vi "LSMcontroller_v66_improvedwfhandling.vi"() -> ()   [LabVIEW 2015] (continued)
                                w2966 = u16 0 items=["unsigned binary", "offset binary", "2's complement"] ("data format (offset binary)")
                                n482 = Initialize Array(sgl 0.0, w2962) -> (w2969:sgl[])
                                n483 = Replace Array Subset(array=w2969, new element=sgl 1.0, index=0) -> (w2967:sgl[])
                                n484 = Reciprocal(x=w2972) -> (1/x=w2973:sgl)
                                n485 = Bundle By Name("Y"=w2967, "dt"=w2973) -> (w2964:waveform(sgl))  [unwired: 1 in]
                                n486 = call-poly <vilib>:"Analog to Digital.vi"("data format (offset binary)"=w2966, "compress digital (T)"=TRUE, "full-scale range (pk-pk)"=1.0, "resolution (16 bit)"=1, "analog waveform"=w2964) -> ("digital waveform"=w2963:digitalwaveform)  [unwired: 3 in, 3 out]
                                }
                                frame True {
                                w2979 = u16 0 items=["unsigned binary", "offset binary", "2's complement"] ("data format (offset binary)")
                                n487 = To Double Precision Float(number=w2982) -> (double precision float=w2989:dbl)
                                n488 = Initialize Array(sgl 0.0, w2982) -> (w2984:sgl[])
                                n489 = Divide(x=w2988, y=w2989) -> (x/y=w2986:dbl)
                                n490 = Round Toward +Infinity(x=w2986) -> (ceil(x): smallest int >= x=w2987:dbl)
                                n491 = Replace Array Subset(array=w2984, new element=sgl 1.0, index=0) -> (w2981:sgl[])
                                n492 = for {
                                N: w2987 -> [_]
                                tunnel: w2981 -> [w2993]
                                tunnel: [w2993] -> w2990 mode=concatenating
                                }
                                n493 = Reciprocal(x=w2991) -> (1/x=w2992:sgl)
                                n494 = Bundle By Name("Y"=w2990, "dt"=w2992) -> (w2977:waveform(sgl))  [unwired: 1 in]
                                n495 = call-poly <vilib>:"Analog to Digital.vi"("data format (offset binary)"=w2979, "compress digital (T)"=TRUE, "full-scale range (pk-pk)"=1.0, "resolution (16 bit)"=1, "analog waveform"=w2977) -> ("digital waveform"=w2976:digitalwaveform)  [unwired: 3 in, 3 out]
                                }
                                }
                                n496 = Build Array (concatenate)(w2951, w2953) -> (w2949:digitalwaveform[])
                                n497 = call "waveformsDObuffer.vi"("DO wf in"=w2949, "command"="set") -> ()  [unwired: 1 out]
                                }
                                frame 2 {
                                n498 = call "waveformsDObuffer.vi"("command"="get") -> ("DO wf out"=w2997:digitalwaveform[])  [unwired: 1 in]
                                n499 = Delete From Array(array=w2997, length=1, index=w3000) -> (deleted portion=w2995:digitalwaveform[], array with subset deleted=w2994:digitalwaveform[])
                                n500 = call "waveformsDObuffer.vi"("DO wf in"=w2994, "command"="set") -> ()  [unwired: 1 out]
                                }
                                frame 3, Default {
                                }
                                frame 0 {
                                n501 = local read "Measurement"() -> (w3003:T4)
                                n502 = To Unsigned Long Integer(number=w3003) -> (unsigned 32bit integer=w3002:u32)
                                n503 = case shown="5..7" w3002 {
                                tunnel: w3004 -> [_ w3007]
                                tunnel: [_ w3006] -> w3001
                                frame 0..4, Default {
                                }
                                frame 5..7 {
                                n504 = call "2pparameters.vi"("command"="get") -> ("params out"=w3014:T10)  [unwired: 1 in]
                                n505 = Unbundle By Name(w3014) -> ("wavdet"=w3015:bool, "sAOxy"=w3017:i32, "refwfsize"=w3018:dbl, "srate Img"=w3016:sgl)
                                n506 = call "waveformsDObuffer.vi"("command"="get") -> ("DO wf out"=w3008:digitalwaveform[])  [unwired: 1 in]
                                n507 = Index Array(array=w3008, index=w3007) -> (element=w3009:digitalwaveform)
                                n508 = case shown="True" w3015 {
                                tunnel: [w3022 w3035] -> w3012
                                tunnel: w3016 -> [w3031 w3050]
                                tunnel: w3017 -> [w3021 w3041]
                                tunnel: w3018 -> [_ w3047]
                                frame False {
                                w3025 = u16 0 items=["unsigned binary", "offset binary", "2's complement"] ("data format (offset binary)")
                                n509 = Initialize Array(sgl 0.0, w3021) -> (w3028:sgl[])
                                n510 = Replace Array Subset(array=w3028, new element=sgl 1.0, index=0) -> (w3026:sgl[])
                                n511 = Reciprocal(x=w3031) -> (1/x=w3032:sgl)
                                n512 = Bundle By Name("Y"=w3026, "dt"=w3032) -> (w3023:waveform(sgl))  [unwired: 1 in]
                                n513 = call-poly <vilib>:"Analog to Digital.vi"("data format (offset binary)"=w3025, "compress digital (T)"=TRUE, "full-scale range (pk-pk)"=1.0, "resolution (16 bit)"=1, "analog waveform"=w3023) -> ("digital waveform"=w3022:digitalwaveform)  [unwired: 3 in, 3 out]
                                }
                                frame True {
                                w3038 = u16 0 items=["unsigned binary", "offset binary", "2's complement"] ("data format (offset binary)")
                                n514 = To Double Precision Float(number=w3041) -> (double precision float=w3048:dbl)
                                n515 = Initialize Array(sgl 0.0, w3041) -> (w3043:sgl[])
                                n516 = Divide(x=w3047, y=w3048) -> (x/y=w3045:dbl)
                                n517 = Round Toward +Infinity(x=w3045) -> (ceil(x): smallest int >= x=w3046:dbl)
                                n518 = Replace Array Subset(array=w3043, new element=sgl 1.0, index=0) -> (w3040:sgl[])
                                n519 = for {
                                N: w3046 -> [_]
                                tunnel: w3040 -> [w3052]
                                tunnel: [w3052] -> w3049 mode=concatenating
                                }
                                n520 = Reciprocal(x=w3050) -> (1/x=w3051:sgl)
                                n521 = Bundle By Name("Y"=w3049, "dt"=w3051) -> (w3036:waveform(sgl))  [unwired: 1 in]
                                n522 = call-poly <vilib>:"Analog to Digital.vi"("data format (offset binary)"=w3038, "compress digital (T)"=TRUE, "full-scale range (pk-pk)"=1.0, "resolution (16 bit)"=1, "analog waveform"=w3036) -> ("digital waveform"=w3035:digitalwaveform)  [unwired: 3 in, 3 out]
                                }
                                }
                                n523 = Build Array(w3009) -> (w3006:digitalwaveform[])
                                n524 = Replace Array Subset(array=w3008, new element=w3012, index=w3007) -> (w3005:digitalwaveform[])
                                n525 = call "waveformsDObuffer.vi"("DO wf in"=w3005, "command"="set") -> ()  [unwired: 1 out]
                                }
                                }
                                }
                                }
                              }
                              frame #10 {
                                n526 = local read "Meastab"() -> (w3067:enum32{"X-Y Image", "Linescan", "Timetrace"})
                                n527 = property on="refwf" class="Ring (strict)"() -> ("RingText.Text"=w3064:string)  [unwired: 2 in, 2 out]
                                n528 = case shown="\"Timetrace\"" w3067 {
                                tunnel: [w3069 w3070] -> w3068
                                frame "X-Y Image", Default {
                                n529 = local read "Sampling rate"() -> (w3069:dbl)
                                }
                                frame "Timetrace" {
                                n530 = local read "srateAODOtt"() -> (w3070:dbl)
                                }
                                }
                                n531 = call "waveformsAObuffer.vi"("command"="get") -> ("AO wf out"=w3055:waveform(dbl)[])  [unwired: 1 in]
                                n532 = local read "wavdet"() -> (w3065:bool)
                                n533 = call "waveformsDObuffer.vi"("command"="get") -> ("DO wf out"=w3059:digitalwaveform[])  [unwired: 1 in]
                                n534 = call "correctwaveformsizetemp.vi"("new sampling frequency (Hz)"=w3068, "start"=TRUE, "reference waveforms to"=w3064, "Analog waveforms in"=w3055, "stop"=FALSE, "Digital waveforms in"=w3059) -> ("analog wf out"=w3061:waveform(dbl)[], "Digital wf out"=w3063:digitalwaveform[], "measpoints"=w3066:i32)
                                n535 = call "GetNumCamFramesv2.vi"("Digital Waveform Graph"=w3063) -> ("Numeric"=w3062:i32)  [unwired: 10 in]
                                n536 = call "waveformsDObuffer.vi"("DO wf in"=w3063, "command"="set") -> ()  [unwired: 1 out]
                                n537 = call "waveformsAObuffer.vi"("AO wf in"=w3061, "command"="set") -> ()  [unwired: 1 out]
                                n538 = local write "Total Camera Frames"(w3062) -> ()
                                n539 = case shown="True" w3065 {
                                tunnel: w3066 -> [_ w3071]
                                frame False {
                                }
                                frame True {
                                n540 = local write "# of frames"(w3071) -> ()
                                }
                                }
                              }
                            }
                          }
                          frame #6 {
                            # "Disabled for conversion to 64 bit"
                            n541 = disable-structure shown="Disabled" {
                              frame Disabled {
                                n542 = local read "Measurement"() -> (w3076:T4)
                                n543 = case shown="\"Lifetime (scan)\"" w3076 {
                                frame "X-Y-t movie", Default {
                                }
                                frame "Lifetime (scan)" {
                                # "total acquisition time"
                                n544 = call "2pparameters.vi"("command"="get") -> ("params out"=w3082:T10)  [unwired: 1 in]
                                n545 = Unbundle By Name(w3082) -> ("measpoints"=w3103:i32, "avpp"=w3104:i32, "sAOxy"=w3083:i32, "srate Img"=w3105:sgl)
                                n546 = Multiply(x=w3103, y=w3104) -> (x*y=w3101:i32)
                                n547 = To Double Precision Float(number=w3083) -> (double precision float=w3088:dbl)
                                n548 = Divide(x=w3088, y=w3105) -> (x/y=w3090:dbl)
                                n549 = To Double Precision Float(number=w3101) -> (double precision float=w3086:dbl)
                                n550 = local read "min phot"() -> (w3097:u32)
                                n551 = local read "expected c/s"() -> (w3098:dbl)
                                n552 = Multiply(x=w3086, y=w3090) -> (x*y=w3084:dbl)
                                n553 = Multiply(x=w3084, y=1000.0) -> (x*y=w3089:dbl)
                                n554 = local read "Ch1 ZeroX"() -> (w3095:i32)
                                n555 = local read "truncate"() -> (w3096:u32)
                                n556 = To Long Integer(number=w3089) -> (32bit integer=w3099:i32)
                                n557 = To Long Integer(number=w3098) -> (32bit integer=w3100:i32)
                                n558 = local read "Number of Bins"() -> (w3091:u32)
                                n559 = local read "Ch1 Level"() -> (w3093:i32)
                                n560 = local read "Ch0 ZeroX"() -> (w3094:i32)
                                n561 = local write "Acquisition time"(w3099) -> ()
                                n562 = local read "Ch0 Level"() -> (w3092:i32)
                                n563 = call "lifetimeparameters.vi"("command"="get") -> ("Params out"=w3080:T19)  [unwired: 1 in]
                                n564 = Add(x=10, y=w3099) -> (x+y=w3087:i32)
                                n565 = Bundle By Name(cluster=w3080, "acq time"=w3087, "acq rate"=w3100, "# bins"=w3091, "Ch0 Level"=w3092, "Ch1 Level"=w3093, "Ch0 ZeroX"=w3094, "Ch1 ZeroX"=w3095, "min photons"=w3097, "truncate"=w3096) -> (w3079:T19)
                                n566 = local write "Acquisition rate"(w3100) -> ()
                                n567 = call "lifetimeparameters.vi"("Params in"=w3079, "command"="set") -> ()  [unwired: 1 out]
                                }
                                }
                                n568 = local read "min phot"() -> (w3074:u32)
                                n569 = Decrement(x=w3074) -> (x-1=w3075:u32)
                                n570 = To Double Precision Float(number=w3075) -> (double precision float=w3073:dbl)
                                n571 = property on="img_CH1" class="IntGraph (strict)"("ZScale.Minimum"=w3073) -> ()  [unwired: 2 in, 2 out]
                              }
                              frame Enabled {
                              }
                            }
                            n572 = local write "64bit disabled"(TRUE ("64bit disabled")) -> ()
                          }
                          frame #7 {
                            n573 = local read "Sampling rate"() -> (w3107:dbl)
                            n574 = call "calcdaqtime.vi"("sampling rate"=w3107) -> ("Calc. time per frame (ms)"=w3106:dbl)
                            n575 = local write "Calc. time per frame (ms)"(w3106) -> ()
                          }
                          frame #8 {
                            n576 = call "2pparameters.vi"("command"="get") -> ("params out"=w3118:T10)  [unwired: 1 in]
                            n577 = local read "Measurement"() -> (w3109:T4)
                            n578 = Unbundle By Name(w3118) -> ("bufferAI"=w3116:i32, "srate"=w3117:sgl)
                            n579 = To Double Precision Float(number=w3116) -> (double precision float=w3110:dbl)
                            n580 = To Double Precision Float(number=w3117) -> (double precision float=w3120:dbl)
                            n581 = case shown="\"X-Y-t movie\", Default" w3109 {
                              tunnel: [w3125 w3129] -> w3108
                              frame "X-Y-t movie", Default {
                                n582 = local read "wavdet"() -> (w3126:bool)
                                n583 = case shown="False" w3126 {
                                tunnel: [w3127 w3128] -> w3125
                                frame False {
                                w3127 = 10123 items=["Finite Samples"=10178, "Continuous Samples"=10123, "Hardware Timed Single Point"=12522] ("sample mode")
                                }
                                frame True {
                                w3128 = 10123 items=["Finite Samples"=10178, "Continuous Samples"=10123, "Hardware Timed Single Point"=12522] ("sample mode")
                                }
                                }
                              }
                              frame "X-Y-Z stack" {
                                w3129 = 10178 items=["Finite Samples"=10178, "Continuous Samples"=10123, "Hardware Timed Single Point"=12522] ("sample mode")
                              }
                            }
                            n584 = Divide(x=w3110, y=w3120) -> (x/y=w3124:dbl)
                            n585 = Multiply(x=w3124, y=2.0) -> (x*y=w3121:dbl)
                            n586 = Max & Min(x=w3121, y=10.0) -> (max(x,y)=w3111:dbl)  [unwired: 1 out]
                            n587 = call "2pparameters.vi"("command"="get") -> ("params out"=w3115:T10)  [unwired: 1 in]
                            n588 = Bundle By Name(cluster=w3115, "timeout"=w3111, "sample mode"=w3108) -> (w3112:T10)
                            n589 = call "2pparameters.vi"("Params in"=w3112, "command"="set") -> ()  [unwired: 1 out]
                          }
                          frame #9 {
                            n590 = local read "# of frames"() -> (w3130:i32)
                            n591 = call "timestamps.vi"("# of frames"=w3130, "command"="init") -> ()  [unwired: 2 in, 1 out]
                          }
                        }
                      }
                      frame #2 {
                        # "Disabled for conversion to 64 bit"
                        n592 = call "prepAO_img.vi"() -> ("Terminal Name with Device Prefix"=w3133:tag)
                        n593 = call "prepAI_img.vi"("triggersource"=w3133) -> ()  [unwired: 2 in]
                        n594 = call "prepCI_img.vi"("ArmStart.DigEdge.Src"=w3133) -> ()  [unwired: 1 in]
                        n595 = call "prepDO_img.vi"() -> ()  [unwired: 2 in]
                        n596 = disable-structure shown="Disabled" {
                          frame Disabled {
                            n597 = local read "Measurement"() -> (w3134:T4)
                            n598 = case shown="\"Lifetime (scan)\"" w3134 {
                              frame "X-Y-t movie", Default {
                              }
                              frame "Lifetime (scan)" {
                                n599 = stacked-sequence {
                                frame #0 {
                                n600 = call "PH-temp.vi"("String"="clear" ("command")) -> ()  [unwired: 2 in, 2 out]
                                n601 = call "PH-temp-raw.vi"("command"="empty") -> ()  [unwired: 1 in, 1 out]
                                }
                                frame #1 {
                                n602 = call "calib.vi"() -> ()  [unwired: 1 in]
                                }
                                frame #2 {
                                n603 = call "setup.vi"() -> ()  [unwired: 1 in]
                                }
                                }
                              }
                            }
                          }
                          frame Enabled {
                          }
                        }
                        n604 = local write "64bit disabled"(TRUE ("64bit disabled")) -> ()
                      }
                      frame #3 {
                        n605 = local read "save\ndata"() -> (w3137:bool)
                        n606 = case shown="True" w3137 {
                          tunnel: w3138 -> [_ w3142]
                          frame False {
                          }
                          frame True {
                            n607 = local read "filename prefix"() -> (w3140:string)
                            n608 = local read "data dir"() -> (w3141:path)
                            n609 = call "preparetiffs.vi"("filename prefix"=w3140, "data dir"=w3141, "timestamp"=w3142) -> ("full-filename"=w3139:string)  [unwired: 1 in]
                            n610 = local write "full-filename"(w3139) -> ()
                          }
                        }
                        n611 = call "preptempbuffers.vi"() -> ()  [unwired: 12 in]
                      }
                      frame #4 {
                        # "Disabled Thorlabs Zstage;\nneeds to be replaced by PI code"
                        n612 = local read "Measurement"() -> (w3143:T4)
                        n613 = case shown="\"X-Y-Z stack\"" w3143 {
                          frame "X-Y-t movie", Default {
                          }
                          frame "X-Y-Z stack" {
                            # "Move Z stage"
                            n614 = stacked-sequence {
                              seq-local: [w3145 _] -> [_ w3158]
                              frame #0 {
                                n615 = local read "Z-Start (um)"() -> (w3149:dbl)
                                n616 = local read "Z-end (um)"() -> (w3148:dbl)
                                n617 = local read "# of frames"() -> (w3150:i32)
                                n618 = call "calcZslice.vi"("current slice"=0, "# of Slices"=w3150, "Z-Start (um)"=w3149, "Z-end (um)"=w3148) -> ("zpos (V)"=w3146:dbl, "zpos (um)"=w3145:dbl)
                                n619 = call "moveZ_V2.vi"("Z"=w3146) -> ()
                                n620 = local write "Cal. Z"(w3145) -> ()
                              }
                              frame #1 {
                                n621 = local read "Pstart"() -> (w3157:dbl)
                                n622 = local read "Pend"() -> (w3156:dbl)
                                n623 = local read "exp?"() -> (w3155:bool)
                                n624 = local read "Z-Start (um)"() -> (w3160:dbl)
                                n625 = local read "Z0"() -> (w3161:dbl)
                                n626 = local read "Z-end (um)"() -> (w3159:dbl)
                                n627 = local read "wavelength(nm)"() -> (w3154:dbl)
                                n628 = local read "# of frames"() -> (w3153:i32)
                                n629 = call "pockelscellzstage.vi"("current slice"=0, "# of Slices"=w3153, "wavelength (nm)"=w3154, "Z0"=w3161, "exp?"=w3155, "Zstart"=w3160, "Pend"=w3156, "Pstart"=w3157, "Z"=w3158, "Zend"=w3159) -> ("T(%)"=w3151:dbl)  [unwired: 1 in]
                                n630 = property on="Laserpower \n(%)" class="Slide (strict)"("Value"=w3151) -> ()  [unwired: 2 in, 2 out]
                                n631 = property on="lpow" class="DigNum (strict)"("Value"=w3151) -> ()  [unwired: 2 in, 2 out]
                              }
                            }
                          }
                        }
                        n632 = local write "Thorlabs Zstage disabled"(TRUE ("64bit disabled")) -> ()
                      }
                      frame #5 {
                        n633 = flat-sequence {
                          frame #0 {
                            n634 = call "2pparameters.vi"("command"="get") -> ("params out"=w3163:T10)  [unwired: 1 in]
                            n635 = Unbundle By Name(w3163) -> ("autoshutter"=w3164:bool)
                            n636 = case shown="True" w3164 {
                              frame False {
                              }
                              frame True {
                                n637 = call "shuttercontrol.vi"("command"="open") -> ()  [unwired: 1 in, 1 out]
                              }
                            }
                          }
                          frame #1 {
                            n638 = call "2pparameters.vi"("command"="get") -> ("params out"=w3168:T10)  [unwired: 1 in]
                            n639 = Tick Count (ms)() -> (millisecond timer value=w3167:u32)
                            n640 = Bundle By Name(cluster=w3168, "starttick"=w3167) -> (w3166:T10)
                            n641 = call "2pparameters.vi"("Params in"=w3166, "command"="set") -> ()  [unwired: 1 out]
                          }
                        }
                      }
                      frame #6 {
                        n642 = local read "Measurement"() -> (w3171:T4)
                        n643 = case shown="\"Lifetime (scan)\"" w3171 {
                          frame "X-Y-t movie" {
                            n644 = flat-sequence {
                              frame #0 {
                                n645 = call "runAI_img.vi"() -> ()  [unwired: 12 in]
                                n646 = call "runCI.vi"() -> ()  [unwired: 12 in]
                                n647 = call "runDO_img.vi"() -> ()  [unwired: 12 in]
                              }
                              frame #1 {
                                n648 = call "runAO_img.vi"() -> ()  [unwired: 12 in]
                              }
                            }
                          }
                          frame "Lifetime (scan)" {
                            # "Disabled for conversion to 64 bit"
                            n649 = disable-structure shown="Disabled" {
                              frame Disabled {
                                n650 = flat-sequence {
                                frame #0 {
                                n651 = call "runLT_img.vi"() -> ()  [unwired: 1 in]
                                n652 = call "runDO_img.vi"() -> ()  [unwired: 12 in]
                                }
                                frame #1 {
                                n653 = call "runAI_img.vi"() -> ()  [unwired: 12 in]
                                n654 = call "runCI.vi"() -> ()  [unwired: 12 in]
                                }
                                frame #2 {
                                n655 = call "runAO_img.vi"() -> ()  [unwired: 12 in]
                                }
                                }
                              }
                              frame Enabled {
                              }
                            }
                            n656 = local write "64bit disabled"(TRUE ("64bit disabled")) -> ()
                          }
                          frame "X-Y-Z stack", Default {
                          }
                        }
                      }
                      frame #7 {
                        # "Disabled for conversion to 64 bit"
                        n657 = while {
                          i -> [w3200]
                          stop <- w3197 stop-if-true
                          n658 = local read "Exit"() -> (w3205:bool)
                          n659 = local read "Stop"() -> (w3196:bool)
                          n660 = Or(x=w3196, y=w3205) -> (x .or. y?=w3201:bool)
                          n661 = case shown="False" w3201 {
                            tunnel: w3200 -> [w3206 _]
                            frame False {
                              n662 = stacked-sequence {
                                seq-local: [w3208 _ _ _ _ _ _] -> [_ _ _ _ _ _ w3337]
                                seq-local: [w3207 _ _ _ _ _ _] -> [_ _ _ _ _ _ w3336]
                                tunnel: w3206 -> [_ w3214 _ _ _ _ _]
                                frame #0 {
                                n663 = local read "Live"() -> (w3209:bool)
                                n664 = case shown="True" w3209 {
                                tunnel: [_ w3211] -> w3208
                                tunnel: [_ w3210] -> w3207
                                frame False {
                                }
                                frame True {
                                n665 = local read "Laserpower \n(%)"() -> (w3210:dbl)
                                n666 = local read "lpow"() -> (w3211:dbl)
                                }
                                }
                                n667 = call "preptempbuffers.vi"() -> ()  [unwired: 12 in]
                                }
                                frame #1 {
                                # "Move in Z if necessary"
                                # "Disabled Thorlabs Zstage;\nneeds to be replaced by PI code"
                                n668 = local read "Measurement"() -> (w3212:T4)
                                n669 = case shown="\"X-Y-Z stack\"" w3212 {
                                tunnel: w3214 -> [_ w3215]
                                frame "X-Y-t movie", Default {
                                }
                                frame "X-Y-Z stack" {
                                n670 = stacked-sequence {
                                seq-local: [w3216 _] -> [_ w3224]
                                tunnel: w3215 -> [w3218 w3223]
                                frame #0 {
                                n671 = local read "Z-Start (um)"() -> (w3220:dbl)
                                n672 = local read "Z-end (um)"() -> (w3219:dbl)
                                n673 = local read "# of frames"() -> (w3221:i32)
                                n674 = call "calcZslice.vi"("current slice"=w3218, "# of Slices"=w3221, "Z-Start (um)"=w3220, "Z-end (um)"=w3219) -> ("zpos (V)"=w3217:dbl, "zpos (um)"=w3216:dbl)
                                n675 = local write "Cal. Z"(w3216) -> ()
                                n676 = call "moveZ_V2.vi"("Z"=w3217) -> ()
                                }
                                frame #1 {
                                n677 = local read "Pstart"() -> (w3229:dbl)
                                n678 = local read "Pend"() -> (w3228:dbl)
                                n679 = local read "exp?"() -> (w3227:bool)
                                n680 = local read "Z-Start (um)"() -> (w3231:dbl)
                                n681 = local read "Z0"() -> (w3232:dbl)
                                n682 = local read "Z-end (um)"() -> (w3230:dbl)
                                n683 = local read "wavelength(nm)"() -> (w3226:dbl)
                                n684 = local read "# of frames"() -> (w3225:i32)
                                n685 = call "pockelscellzstage.vi"("current slice"=w3223, "# of Slices"=w3225, "wavelength (nm)"=w3226, "Z0"=w3232, "exp?"=w3227, "Zstart"=w3231, "Pend"=w3228, "Pstart"=w3229, "Z"=w3224, "Zend"=w3230) -> ("T(%)"=w3222:dbl)  [unwired: 1 in]
                                n686 = property on="Laserpower \n(%)" class="Slide (strict)"("Value"=w3222) -> ()  [unwired: 2 in, 2 out]
                                n687 = property on="lpow" class="DigNum (strict)"("Value"=w3222) -> ()  [unwired: 2 in, 2 out]
                                }
                                }
                                }
                                }
                                n688 = local write "Thorlabs Zstage disabled"(TRUE ("64bit disabled")) -> ()
                                }
                                frame #2 {
                                # "main loop"
                                n689 = for {
                                N: "avpp" -> [_]
                                i -> [w3238]
                                n690 = local read "Stop"() -> (w3236:bool)
                                n691 = local read "Exit"() -> (w3235:bool)
                                n692 = Increment(x=w3238) -> (x+1=w3237:i32)
                                n693 = Or(x=w3236, y=w3235) -> (x .or. y?=w3234:bool)
                                n694 = case shown="False" w3234 {
                                tunnel: w3237 -> [w3239 _]
                                frame False {
                                n695 = stacked-sequence {
                                seq-local: [w3240 _ _ _ _ _ _] -> [_ _ _ w3253 w3265 w3273 _]
                                tunnel: w3239 -> [w3241 _ _ _ _ _ _]
                                frame #0 {
                                n696 = local read "Live"() -> (w3240:bool)
                                n697 = case shown="True" w3240 {
                                tunnel: w3241 -> [_ w3244]
                                frame False {
                                }
                                frame True {
                                # "collect timetag for current image\nplus curent average"
                                n698 = To Single Precision Float(number=w3244) -> (single precision float=w3242:sgl)
                                n699 = Tick Count (ms)() -> (millisecond timer value=w3243:u32)
                                n700 = local write "Tick for Frame"(w3243) -> ()
                                n701 = local write "Current Average"(w3242) -> ()
                                }
                                }
                                }
                                frame #1 {
                                n702 = local read "Measurement"() -> (w3245:T4)
                                n703 = case shown="\"X-Y-Z stack\"" w3245 {
                                frame "X-Y-t movie", Default {
                                }
                                frame "X-Y-Z stack" {
                                n704 = stacked-sequence {
                                frame #0 {
                                n705 = disable-structure shown="Disabled" {
                                frame Disabled {
                                n706 = call "2pparameters.vi"("command"="get") -> ("params out"=w3247:T10)  [unwired: 1 in]
                                n707 = Unbundle By Name(w3247) -> ("autoshutter"=w3248:bool)
                                n708 = case shown="True" w3248 {
                                frame False {
                                }
                                frame True {
                                n709 = call "shuttercontrol.vi"("command"="open") -> ()  [unwired: 1 in, 1 out]
                                }
                                }
                                }
                                frame Enabled {
                                }
                                }
                                }
                                frame #1 {
                                n710 = call "runAI_img.vi"() -> ()  [unwired: 12 in]
                                n711 = call "runCI.vi"() -> ()  [unwired: 12 in]
                                n712 = call "runDO_img.vi"() -> ()  [unwired: 12 in]
                                }
                                frame #2 {
                                n713 = call "runAO_img.vi"() -> ()  [unwired: 12 in]
                                }
                                }
                                }
                                }
                                }
                                frame #2 {
                                n714 = call "collectCI_img.vi"() -> ("Avg cts/s"=w3252:dbl, "recorded samples"=w3251:i32)  [unwired: 1 out]
                                n715 = call "collectAI_img.vi"() -> ("wrap"=w3250:i32)  [unwired: 3 in]
                                n716 = local write "scol"(w3251) -> ()
                                n717 = local write "wrap"(w3250) -> ()
                                n718 = local write "Avg Counts/s"(w3252) -> ()
                                }
                                frame #3 {
                                n719 = case shown="True" w3253 {
                                frame False {
                                }
                                frame True {
                                n720 = local read "Measurement"() -> (w3254:T4)
                                n721 = case shown="\"X-Y-t movie\", Default" w3254 {
                                frame "X-Y-t movie", Default {
                                n722 = local read "ROI Type"() -> (w3255:u16)
                                n723 = case shown="0" w3255 {
                                frame 0 {
                                # "display chosen channels"
                                n724 = local read "Current Average"() -> (w3264:sgl)
                                n725 = local read "image1list"() -> (w3260:u16)
                                n726 = local read "image2list"() -> (w3263:u16)
                                n727 = To Unsigned Word Integer(number=w3263) -> (unsigned 16bit integer=w3258:u16)
                                n728 = To Unsigned Word Integer(number=w3260) -> (unsigned 16bit integer=w3259:u16)
                                n729 = call "dattoimage.vi"("image2list"=w3258, "Current Average"=w3264, "image1list"=w3259) -> ("image 2 array out"=w3262:sgl[][], "image 1 array out"=w3261:sgl[][])
                                n730 = Transpose 2D Array(2D array=w3261) -> (transposed array=w3257:sgl[][])
                                n731 = Transpose 2D Array(2D array=w3262) -> (transposed array=w3256:sgl[][])
                                n732 = local write "img_CH1"(w3257) -> ()
                                n733 = local write "img_CH2"(w3256) -> ()
                                }
                                frame 1, Default {
                                }
                                }
                                }
                                frame "Lifetime (scan)" {
                                }
                                }
                                }
                                }
                                }
                                frame #4 {
                                n734 = case shown="True" w3265 {
                                frame False {
                                }
                                frame True {
                                # "set colormaps"
                                n735 = call "misc-global.vi"("command"="get") -> ("misc out"=w3269:cluster{"Colormaps":u32[][]})  [unwired: 1 in]
                                n736 = Unbundle By Name(w3269) -> ("Colormaps"=w3268:u32[][])
                                n737 = control-ref of="img_CH1"() -> (w3272:refnum<vi>)
                                n738 = control-ref of="img_CH2"() -> (w3271:refnum<vi>)
                                n739 = Index Array(array=w3268, index (row)="Colormap") -> (element=w3267:u32[])  [unwired: 1 in]
                                n740 = property class="IntGraph (strict)"(reference=w3272, "Color Table"=w3267) -> ()  [unwired: 1 in, 2 out]
                                n741 = property class="IntGraph (strict)"(reference=w3271, "Color Table"=w3267) -> ()  [unwired: 1 in, 2 out]
                                }
                                }
                                }
                                frame #5 {
                                n742 = case shown="True" w3273 {
                                frame False {
                                }
                                frame True {
                                # "crude estimate of time per frame\n(resolution is 1 ms), not so much for\nplotting purposes, more for debugging\ncollection and processing data"
                                n743 = local read "ypixels ref"() -> (w3278:i32)
                                n744 = local read "Tick for Frame"() -> (w3279:u32)
                                n745 = Tick Count (ms)() -> (millisecond timer value=w3280:u32)
                                n746 = To Double Precision Float(number=w3278) -> (double precision float=w3277:dbl)
                                n747 = Subtract(x=w3280, y=w3279) -> (x-y=w3275:u32)
                                n748 = To Double Precision Float(number=w3275) -> (double precision float=w3276:dbl)
                                n749 = local write "Meas. time per frame (ms)"(w3275) -> ()
                                n750 = Divide(x=w3276, y=w3277) -> (x/y=w3274:dbl)
                                n751 = local write "time per line (ms)"(w3274) -> ()
                                }
                                }
                                }
                                frame #6 {
                                n752 = local read "Measurement"() -> (w3281:T4)
                                n753 = case shown="\"X-Y-Z stack\"" w3281 {
                                frame "X-Y-t movie", Default {
                                }
                                frame "X-Y-Z stack" {
                                n754 = call "2pparameters.vi"("command"="get") -> ("params out"=w3283:T10)  [unwired: 1 in]
                                n755 = Unbundle By Name(w3283) -> ("autoshutter"=w3284:bool)
                                n756 = call "stopCI_img.vi"() -> ()  [unwired: 12 in]
                                n757 = call "stopAI_img.vi"() -> ()  [unwired: 12 in]
                                n758 = case shown="True" w3284 {
                                frame False {
                                }
                                frame True {
                                n759 = call "shuttercontrol.vi"("command"="close") -> ()  [unwired: 1 in, 1 out]
                                }
                                }
                                n760 = Wait (ms)(milliseconds to wait=u32 100) -> ()  [unwired: 1 out]
                                n761 = call "stopAO_img.vi"() -> ()  [unwired: 12 in]
                                n762 = call "stopDO_img.vi"() -> ()  [unwired: 12 in]
                                }
                                }
                                }
                                }
                                }
                                frame True {
                                }
                                }
                                }
                                }
                                frame #3 {
                                n763 = local read "Measurement"() -> (w3287:T4)
                                n764 = case shown="\"Lifetime (scan)\"" w3287 {
                                frame "X-Y-t movie", Default {
                                }
                                frame "Lifetime (scan)" {
                                w3290 = u16 2 items=["Stream to disk", "Post process", "real time process"] ("Ring")
                                n765 = local read "T3R Data processing"() -> (w3291:u16)
                                n766 = Equal?(x=w3291, y=w3290) -> (x = y?=w3289:bool)
                                n767 = case shown="True" w3289 {
                                frame False {
                                }
                                frame True {
                                n768 = disable-structure shown="Disabled" {
                                frame Disabled {
                                n769 = local read "lineshift"() -> (w3294:i32)
                                n770 = call "wrapcutlifetime.vi"("lineshift"=w3294) -> ("pt3img"=w3296:u16[][], "lifetimes"=w3295:sgl[][], "okay"=w3292:bool, "# of frames"=w3293:i32)
                                n771 = case shown="True" w3292 {
                                tunnel: w3296 -> [_ w3306]
                                tunnel: w3295 -> [_ w3304]
                                tunnel: w3293 -> [_ w3300]
                                frame False {
                                }
                                frame True {
                                # "lifetime"
                                # "intensity"
                                n772 = Transpose 2D Array(2D array=w3306) -> (transposed array=w3298:u16[][])
                                n773 = Transpose 2D Array(2D array=w3304) -> (transposed array=w3305:sgl[][])
                                n774 = local write "frames recorded"(w3300) -> ()
                                n775 = local read "counts"() -> (w3299:i32)
                                n776 = Array Max & Min(array=w3298) -> (max value=w3303:u16)  [unwired: 3 out]
                                n777 = To Single Precision Float(number=w3298) -> (single precision float=w3297:sgl[][])
                                n778 = local write "img_CH2"(w3305) -> ()
                                n779 = local write "img_CH1"(w3297) -> ()
                                n780 = Quotient & Remainder(x=w3299, y=w3300) -> (floor(x/y)=→"photons/frame":i32)  [unwired: 1 out]
                                n781 = To Double Precision Float(number=w3303) -> (double precision float=w3302:dbl)
                                n782 = property on="img_CH1" class="IntGraph (strict)"("ZScale.Maximum"=w3302) -> ()  [unwired: 2 in, 2 out]
                                }
                                }
                                }
                                frame Enabled {
                                }
                                }
                                }
                                }
                                }
                                }
                                n783 = local read "save\ndata"() -> (w3288:bool)
                                n784 = case shown="True" w3288 {
                                frame False {
                                }
                                frame True {
                                n785 = local read "Current Average"() -> (w3307:sgl)
                                n786 = call "savetiffs.vi"("current average"=w3307) -> ()
                                }
                                }
                                }
                                frame #4 {
                                n787 = local read "save\ndata"() -> (w3308:bool)
                                n788 = case shown="True" w3308 {
                                frame False {
                                }
                                frame True {
                                n789 = local read "points recorded"() -> (w3310:i32)
                                n790 = call "timestamps.vi"("points recorded"=w3310, "command"="add") -> ()  [unwired: 2 in, 1 out]
                                }
                                }
                                }
                                frame #5 {
                                n791 = local read "Live"() -> (w3311:bool)
                                n792 = case shown="True" w3311 {
                                frame False {
                                }
                                frame True {
                                n793 = local read "downright"() -> (w3316:bool)
                                n794 = local read "downleft"() -> (w3318:bool)
                                n795 = local read "upright"() -> (w3314:bool)
                                n796 = local read "upleft"() -> (w3312:bool)
                                n797 = local read "down"() -> (w3317:bool)
                                n798 = local read "right"() -> (w3315:bool)
                                n799 = local read "left"() -> (w3319:bool)
                                n800 = local read "up"() -> (w3313:bool)
                                n801 = Compound Arithmetic op=OR(w3312, w3313, w3314, w3315, w3316, w3317, w3318, w3319) -> (w3320:bool)
                                n802 = case shown="True" w3320 {
                                frame False {
                                }
                                frame True {
                                n803 = stacked-sequence {
                                frame #0 {
                                n804 = local read "downright"() -> (w3322:bool)
                                n805 = local read "downleft"() -> (w3324:bool)
                                n806 = local read "BigSmall"() -> (w3321:bool)
                                n807 = local read "upright"() -> (w3326:bool)
                                n808 = local read "upleft"() -> (w3329:bool)
                                n809 = local read "down"() -> (w3325:bool)
                                n810 = local read "right"() -> (w3327:bool)
                                n811 = local read "left"() -> (w3323:bool)
                                n812 = local read "up"() -> (w3328:bool)
                                n813 = call "movestageparams.vi"("command"="get") -> ("Params out"=w3332:T20)  [unwired: 1 in]
                                n814 = Bundle By Name(cluster=w3332, "upleft"=w3329, "up"=w3328, "upright"=w3326, "right"=w3327, "downright"=w3322, "down"=w3325, "downleft"=w3324, "left"=w3323, "Bigsmall"=w3321) -> (w3333:T20)
                                n815 = call "movestageparams.vi"("Params in"=w3333, "command"="set") -> ()  [unwired: 1 out]
                                }
                                frame #1 {
                                n816 = call "movestage.vi"() -> ()  [unwired: 12 in]
                                }
                                frame #2 {
                                w3334 = FALSE ("OK Button")
                                w3335 = FALSE ("OK Button")
                                n817 = property on="down" class="Bool (strict)"("Value"=w3335) -> ()  [unwired: 2 in, 2 out]
                                n818 = property on="up" class="Bool (strict)"("Value"=w3335) -> ()  [unwired: 2 in, 2 out]
                                n819 = property on="right" class="Bool (strict)"("Value"=w3335) -> ()  [unwired: 2 in, 2 out]
                                n820 = property on="left" class="Bool (strict)"("Value"=w3335) -> ()  [unwired: 2 in, 2 out]
                                n821 = property on="upright" class="Bool (strict)"("Value"=w3334) -> ()  [unwired: 2 in, 2 out]
                                n822 = property on="downleft" class="Bool (strict)"("Value"=w3334) -> ()  [unwired: 2 in, 2 out]
                                n823 = property on="downright" class="Bool (strict)"("Value"=w3334) -> ()  [unwired: 2 in, 2 out]
                                n824 = property on="upleft" class="Bool (strict)"("Value"=w3334) -> ()  [unwired: 2 in, 2 out]
                                }
                                }
                                }
                                }
                                }
                                }
                                }
                                frame #6 {
                                n825 = local read "Live"() -> (w3338:bool)
                                n826 = case shown="True" w3338 {
                                tunnel: w3337 -> [_ w3345]
                                tunnel: w3336 -> [_ w3344]
                                frame False {
                                }
                                frame True {
                                n827 = local read "Laserpower \n(%)"() -> (w3340:dbl)
                                n828 = local read "lpow"() -> (w3339:dbl)
                                n829 = Not Equal?(x=w3339, y=w3345) -> (x != y?=w3341:bool)
                                n830 = Not Equal?(x=w3340, y=w3344) -> (x != y?=w3342:bool)
                                n831 = Or(x=w3342, y=w3341) -> (x .or. y?=w3343:bool)
                                n832 = case shown="True" w3343 {
                                tunnel: w3342 -> [_ w3349]
                                tunnel: w3341 -> [_ w3348]
                                tunnel: w3340 -> [_ w3347]
                                tunnel: w3339 -> [_ w3346]
                                frame False {
                                }
                                frame True {
                                n833 = case shown="True" w3349 {
                                tunnel: w3347 -> [_ w3352]
                                frame False {
                                }
                                frame True {
                                n834 = local read "wavelength(nm)"() -> (w3353:dbl)
                                n835 = call "setpockelscellT.vi"("wavelength(nm)"=w3353, "transmission"=w3352) -> ()  [unwired: 1 in]
                                n836 = property on="lpow" class="DigNum (strict)"("Value"=w3352) -> ()  [unwired: 2 in, 2 out]
                                }
                                }
                                n837 = case shown="True" w3348 {
                                tunnel: w3346 -> [_ w3350]
                                frame False {
                                }
                                frame True {
                                n838 = local read "wavelength(nm)"() -> (w3351:dbl)
                                n839 = call "setpockelscellT.vi"("wavelength(nm)"=w3351, "transmission"=w3350) -> ()  [unwired: 1 in]
                                n840 = property on="Laserpower \n(%)" class="Slide (strict)"("Value"=w3350) -> ()  [unwired: 2 in, 2 out]
                                }
                                }
                                }
                                }
                                }
                                }
                                }
                              }
                            }
                            frame True {
                            }
                          }
                          n841 = Increment(x=w3200) -> (x+1=w3199:i32)
                          "points recorded" <- w3199
                          n842 = call "stopcond.vi"("prec"=w3199) -> ("stop"=w3198:bool)
                          n843 = local read "Stop"() -> (w3204:bool)
                          n844 = local read "Exit"() -> (w3203:bool)
                          n845 = Or(x=w3204, y=w3203) -> (x .or. y?=w3202:bool)
                          n846 = Or(x=w3198, y=w3202) -> (x .or. y?=w3197:bool)
                        }
                        n847 = disable-structure shown="Disabled" {
                          disable-tunnel: w3174 -> [w3180 _]
                          frame Disabled {
                            w3177 = u16 0 items=["Stream to disk", "Post process", "real time process"] ("Ring")
                            n848 = local read "T3R Data processing"() -> (w3176:u16)
                            n849 = Equal?(x=w3176, y=w3177) -> (x = y?=w3175:bool)
                            n850 = local read "save\ndata"() -> (w3179:bool)
                            n851 = local read "Measurement"() -> (w3181:T4)
                            n852 = And(x=w3179, y=w3175) -> (x .and. y?=w3178:bool)
                            n853 = case shown="\"Lifetime (scan)\"" w3181 {
                              tunnel: w3180 -> [_ w3185]
                              tunnel: w3178 -> [_ w3184]
                              frame "X-Y-t movie", Default {
                              }
                              frame "Lifetime (scan)" {
                                n854 = case shown="True" w3184 {
                                selector: w3184 -> [w3186 w3191]
                                tunnel: w3185 -> [_ w3189]
                                tunnel: [path "" ("appended path") w3192] -> w3183
                                tunnel: [w3186 w3191] -> w3182
                                frame False {
                                }
                                frame True {
                                n855 = local read "filename prefix"() -> (w3190:string)
                                n856 = local read "data dir"() -> (w3193:path)
                                n857 = call "generatedatafilename.vi"("timestamp"=w3189, "filename prefix in"=w3190) -> ("full-filename"=w3188:string)
                                n858 = Concatenate Strings(w3188, ".lvpt3img" ("string")) -> (w3195:string)
                                n859 = Build Path(base path=w3193, name or relative path=w3195) -> (appended path=w3192:path)
                                }
                                }
                                n860 = call "collectLT_img_v2.vi"("stream?"=w3182, "data file"=w3183) -> ()  [unwired: 2 out]
                              }
                            }
                          }
                          frame Enabled {
                          }
                        }
                        n861 = local write "64bit disabled"(TRUE ("64bit disabled")) -> ()
                      }
                      frame #8 {
                        # "Disabled for conversion to 64 bit"
                        n862 = local read "Measurement"() -> (w3356:T4)
                        n863 = case shown="\"Lifetime (scan)\"" w3356 {
                          tunnel: w3355 -> [_ _ w3357]
                          frame "X-Y-t movie", Default {
                          }
                          frame "X-Y-Z stack" {
                            n864 = call "eraseDO_img.vi"() -> ()  [unwired: 12 in]
                            n865 = call "eraseAO_img.vi"() -> ()  [unwired: 12 in]
                            n866 = call "eraseCI_img.vi"() -> ()  [unwired: 12 in]
                            n867 = call "eraseAI_img.vi"() -> ()  [unwired: 12 in]
                          }
                          frame "Lifetime (scan)" {
                            n868 = disable-structure shown="Disabled" {
                              disable-tunnel: w3357 -> [w3358 _]
                              frame Disabled {
                                n869 = stacked-sequence {
                                tunnel: w3358 -> [_ _ w3372 _ _]
                                frame #0 {
                                n870 = disable-structure shown="Disabled" {
                                frame Disabled {
                                n871 = call "stoperaseCI.vi"() -> ()  [unwired: 12 in]
                                n872 = call "stoperaseDO_img.vi"() -> ()  [unwired: 12 in]
                                n873 = call "stoperaseAO_img.vi"() -> ()  [unwired: 12 in]
                                n874 = call "stoperaseAI_img.vi"() -> ()  [unwired: 12 in]
                                }
                                frame Enabled {
                                }
                                }
                                }
                                frame #1 {
                                n875 = disable-structure shown="Disabled" {
                                frame Disabled {
                                n876 = local read "Acquisition time"() -> (w3362:i32)
                                n877 = call "collect_allLT_img.vi"() -> ("counts"=w3364:i32)  [unwired: 1 out]
                                n878 = local read "counts"() -> (w3365:i32)
                                n879 = Add(x=w3365, y=w3364) -> (x+y=w3363:i32)
                                "counts" <- w3363
                                n880 = Divide(x=w3363, y=w3362) -> (x/y=w3361:dbl)
                                n881 = Multiply(x=1000.0, y=w3361) -> (x*y=w3360:dbl)
                                n882 = local write "Avg Counts/s"(w3360) -> ()
                                }
                                frame Enabled {
                                }
                                }
                                }
                                frame #2 {
                                w3368 = u16 0 items=["Stream to disk", "Post process", "real time process"] ("Ring")
                                n883 = local read "T3R Data processing"() -> (w3367:u16)
                                n884 = local read "save\ndata"() -> (w3370:bool)
                                n885 = Equal?(x=w3367, y=w3368) -> (x = y?=w3366:bool)
                                n886 = Not(x=w3366) -> (.not. x?=w3371:bool)
                                n887 = And(x=w3370, y=w3371) -> (x .and. y?=w3369:bool)
                                n888 = case shown="True" w3369 {
                                tunnel: w3372 -> [_ w3374]
                                frame False {
                                }
                                frame True {
                                n889 = local read "filename prefix"() -> (w3375:string)
                                n890 = local read "data dir"() -> (w3380:path)
                                n891 = call "2pparameters.vi"("command"="get") -> ("params out"=w3395:T10)  [unwired: 1 in]
                                n892 = call "generatedatafilename.vi"("timestamp"=w3374, "filename prefix in"=w3375) -> ("full-filename"=w3373:string)
                                n893 = Unbundle By Name(w3395) -> ("srate"=w3393:sgl, "sAOxy"=w3392:i32, "Xpixels Img"=w3390:i32, "Ypixels Img"=w3388:i32)
                                n894 = Concatenate Strings(w3373, ".lvpt3img" ("string")) -> (w3378:string)
                                n895 = Build Path(base path=w3380, name or relative path=w3378) -> (appended path=w3377:path)
                                n896 = To Unsigned Long Integer(number=w3393) -> (unsigned 32bit integer=w3394:u32)
                                n897 = To Unsigned Long Integer(number=w3392) -> (unsigned 32bit integer=w3391:u32)
                                n898 = To Unsigned Long Integer(number=w3390) -> (unsigned 32bit integer=w3389:u32)
                                n899 = To Unsigned Long Integer(number=w3388) -> (unsigned 32bit integer=w3387:u32)
                                n900 = call "PH-temp-raw.vi"("command"="get") -> ("array out"=w3386:u32[])  [unwired: 1 in]
                                n901 = Build Array (concatenate)(w3394, w3391, w3389, w3387, w3386) -> (w3385:u32[])
                                n902 = Open/Create/Replace File(file path (use dialog)=w3377, operation (0:open)=T8."replace or create") -> (refnum out=w3384:refnum<file>, error out=w3383:errorcluster)  [unwired: 4 in, 1 out]
                                n903 = Write to Binary File(file (use dialog)=w3384, data=w3385, error in=w3383, 5:FALSE ("prepend array or string size? (T)")) -> (refnum out=w3381:refnum<file>, error out=w3382:errorcluster)  [unwired: 2 in, 1 out]
                                n904 = Close File(refnum=w3381, error in=w3382) -> ()  [unwired: 2 out]
                                }
                                }
                                n905 = call "stoperaseLT_img.vi"() -> ()  [unwired: 1 in]
                                }
                                frame #3 {
                                w3401 = u16 1 items=["Stream to disk", "Post process", "real time process"] ("Ring")
                                n906 = local read "T3R Data processing"() -> (w3400:u16)
                                n907 = Equal?(x=w3400, y=w3401) -> (x = y?=w3399:bool)
                                n908 = case shown="True" w3399 {
                                frame False {
                                }
                                frame True {
                                # "intensity"
                                # "lifetime"
                                # "intensity"
                                n909 = property on="img_CH1" class="IntGraph (strict)"() -> ("Value"=w3414:sgl[][])  [unwired: 2 in, 2 out]
                                n910 = Array Max & Min(array=w3414) -> (max value=w3415:sgl)  [unwired: 3 out]
                                n911 = local read "lineshift"() -> (w3402:i32)
                                n912 = local read "min phot"() -> (w3416:u32)
                                n913 = To Unsigned Long Integer(number=w3415) -> (unsigned 32bit integer=w3418:u32)
                                n914 = local read "counts"() -> (w3404:i32)
                                n915 = call "wrapcutlifetime.vi"("lineshift"=w3402) -> ("pt3img"=w3413:u16[][], "lifetimes"=w3411:sgl[][], "okay"=w3406:bool, "# of frames"=w3403:i32)
                                "frames recorded" <- w3403
                                n916 = Greater?(x=w3416, y=w3418) -> (0:w3417:bool)
                                n917 = Quotient & Remainder(x=w3404, y=w3403) -> (floor(x/y)=w3405:i32)  [unwired: 1 out]
                                n918 = Transpose 2D Array(2D array=w3413) -> (transposed array=w3407:u16[][])
                                n919 = Transpose 2D Array(2D array=w3411) -> (transposed array=w3412:sgl[][])
                                n920 = And(x=w3417, y=w3406) -> (x .and. y?=w3419:bool)
                                n921 = local write "img_CH2"(w3412) -> ()
                                n922 = local write "photons/frame"(w3405) -> ()
                                n923 = Array Max & Min(array=w3407) -> (max value=w3408:u16)  [unwired: 3 out]
                                n924 = To Single Precision Float(number=w3407) -> (single precision float=w3410:sgl[][])
                                n925 = case shown="True" w3419 {
